vi "air_humidity_calculate.vi"(11 "Numeric in":dbl) -> (3 "Numeric out":dbl)   [LabVIEW 2014]
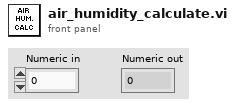
[diagram p1: front panel]
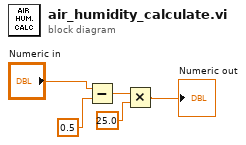
[diagram p0: block diagram]
diagram:
  n1 = Subtract(x="Numeric in", y=0.5) -> (x-y=w3:dbl)
  n2 = Multiply(x=w3, y=25.0) -> (x*y=→"Numeric out":dbl)
